vi "tearDown.vi"(8 "error in (no error)":errorcluster, 11 "reference in":refnum<class "Add User.lvclass">) -> (0 "error out":errorcluster, 3 "reference out":refnum<class "Add User.lvclass">)   [LabVIEW 2017, in "Add User.lvclass"]
doc: "tearDown runs after the test method has completed. Use this method to clean up any operations or references that were opened by setUp or the test method. Unit tests should be independent of other unit tests so this VI should ensure that the next test can run in a 'clean' test environment."
uses:
  Add User.lvclass
  Add User.lvclass/Add User.ctl
  Source/User Configuration Manager Ref/By Ref.lvlib
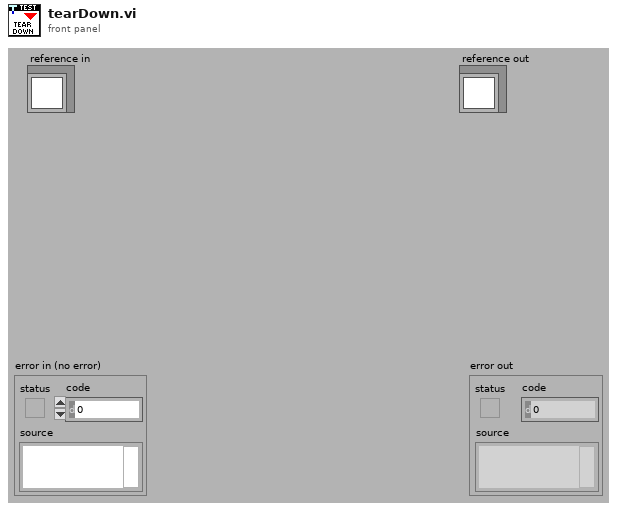
[diagram p1: front panel]
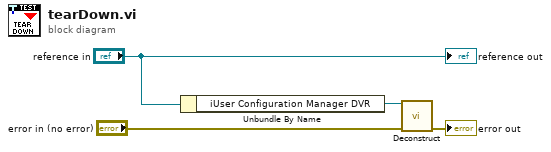
[diagram p0: block diagram]
diagram:
  n1 = Unbundle By Name("reference in") -> ("iUser Configuration Manager DVR"=w2:refnum<data-value>)
  n2 = call "Deconstruct.vi"("iUser Configuration Manager DVR"=w2, "Error In"="error in (no error)") -> ("Error Out"=→"error out":errorcluster)  [unwired: 13 in]
  "reference out" <- "reference in"
